vi "Config LocalSync.vi"(8 "error in (no error)":errorcluster, 11 "Dir":path) -> (0 "error out":errorcluster, 3 "Protocol out":refnum<class "Protocol.lvclass">)   [LabVIEW 2020, in "CSM-FileSync.lvlib"]
uses:
  CSM-FileSync.lvlib
  _fileSync_Support/Base/Protocol/Protocol.lvclass
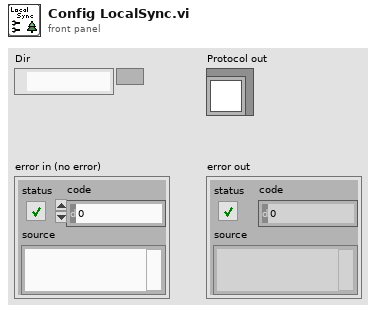
[diagram p1: front panel]
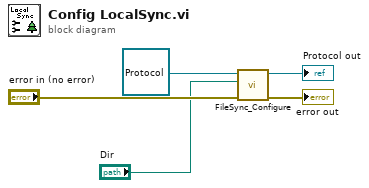
[diagram p0: block diagram]
diagram:
  n1 = call "FileSync_Configure.vi"("error in (no error)"="error in (no error)", "Dir"="Dir", "Protocol in"=refnum<class "Protocol.lvclass"> refnum ("FileSync -- Base.lvlib:Protocol.lvclass")) -> ("error out"=→"error out":errorcluster, "Protocol out"=→"Protocol out":refnum<class "Protocol.lvclass">)  [unwired: 7 in]
